vi "Log_PACKET Receive State Machine_FORMAT.vi"(8 "Evals in a row":i32, 9 "Complete Packet":T1 {"Packet Data" format="%.0x"}, 10 "New Packet Data":u8[](array[numeric]), 11 "Packet Data WIP":u8[](array[numeric])) -> (2 "resulting string":string)   [LabVIEW 2014]
uses:
  PacketMode/SRV_PM_Packet.ctl
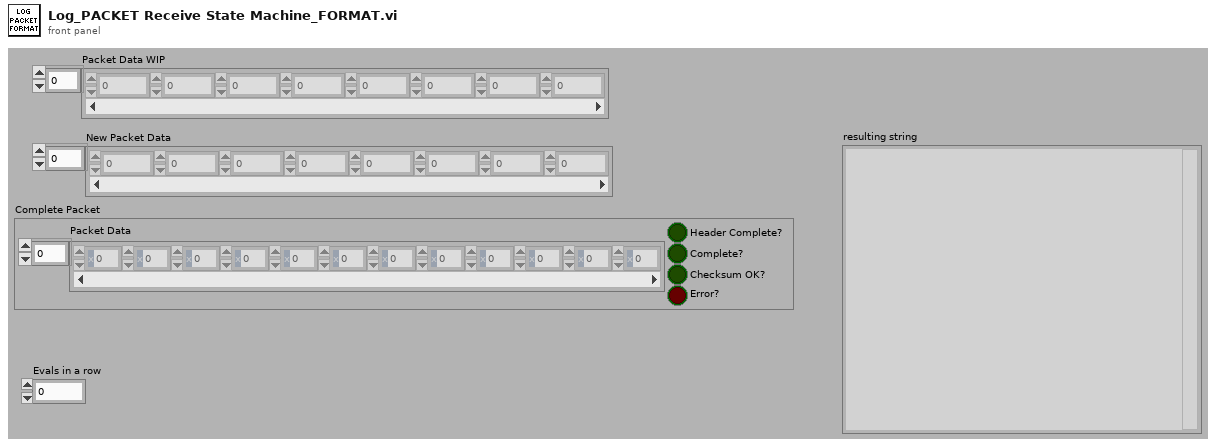
[diagram p1: front panel]
types:
  T1 = typedef "SRV_PM_Packet.ctl" = cluster{"Packet Data":u8[], "Header Complete?":bool, "Complete?":bool, "Checksum OK?":bool, "Error?":bool}
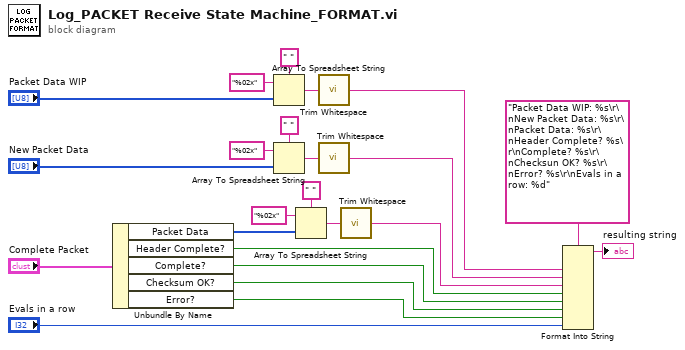
[diagram p0: block diagram]
diagram:
  n1 = Unbundle By Name("Complete Packet") -> ("Packet Data"=w12:u8[], "Header Complete?"=w6:bool, "Complete?"=w5:bool, "Checksum OK?"=w4:bool, "Error?"=w3:bool)
  n2 = Array To Spreadsheet String(delimiter (Tab)=" ", array="Packet Data WIP", 3:"%02x" ("format string")) -> (spreadsheet string=w20:string)
  n3 = Array To Spreadsheet String(delimiter (Tab)=" ", array="New Packet Data", 3:"%02x" ("format string")) -> (spreadsheet string=w19:string)
  n4 = Array To Spreadsheet String(delimiter (Tab)=" ", array=w12, 3:"%02x" ("format string")) -> (spreadsheet string=w11:string)
  n5 = call <vilib>:"Trim Whitespace.vi"("string"=w20) -> ("trimmed string"=w9:string)  [unwired: 1 in]
  n6 = call <vilib>:"Trim Whitespace.vi"("string"=w19) -> ("trimmed string"=w8:string)  [unwired: 1 in]
  n7 = call <vilib>:"Trim Whitespace.vi"("string"=w11) -> ("trimmed string"=w7:string)  [unwired: 1 in]
  n8 = Format Into String(format string="Packet Data WIP: %s\r\nNew Packet Data: %s\r\nPacket Data: %s\r\nHeader Complete? %s\r\nComplete? %s\r\nChecksun OK? %s\r\nError? %s\r\nEvals in a row: %d", w9, w8, w7, w6, w5, w4, w3, "Evals in a row") -> (resulting string=→"resulting string":string)  [unwired: 2 in, 1 out]
